vi "Bilateral_Filter.vi"() -> ()   [LabVIEW 2019]
doc: "This demo illustrates the grayscale morphological operations on grayscale images.\n\nOUTPUT:\nThe output of this demo displays the original grayscale image and the result of applying the grayscale morphological operation.\n\nSPECIAL EXAMPLES:\nSelect \"Images/Noisy-Images/Eggs-S&P90%.tif\" image for the following examples. This is an image corrupted by Salt and Pepper noise.\n\nDilation: Increasing the windows size from N=3 to N=25 increases peaks and decreases the size of valleys in the image. This is clear by seeing that the black noisy pixels vanish, while the white noisy pixels increase in size. The shape of the window can be seen at isolated white pixels illustrating an \"impulse reponse\" (try a cross shaped filter).\n\nErosion: Increasing the window size from N=3 to N=25 erodes/removes peaks (bright regions) and increases valleys (dark regions). The shape of the window can be seen at isolated dark pixels illustrating an \"impulse reponse\" (try a cross shaped filter).\n\nMedian (Majority): Possess attributes of both Dilation and Erosion operators - i.e. removes small black and white regions without changing the size of large objects. This option runs slower since the pixels have to be sorted first. \n\nClose: This operation removes small black objects, but does not change the size of the signal (like Dilation/Erosion). \n\nOpen: This operation removes small white objects, but does not change the size of the signal (like Dilation/Erosion).\n\nClose-Open (and Open-Close): This operation is very similar to the Median in its performance. However, there is an intense smoothing of the image, when compared to the Median filter."
uses:
  <vilib>/vision/NI_Vision_Development_Module.lvlib
panel:
  in  "SigmaS 2":dbl=1.0 format="%.2f"
  in  "sigma copy 2":dbl format="%.2f"
  in  "SigmaI":dbl=1.0 format="%.2f"
  in  "sigma copy":dbl format="%.2f"
  in  "SigmaS":dbl=1.0 format="%.2f"
  in  "STOP":bool
  in  "Window Shape copy":T1(ring)
  in  "Window Shape":T1(ring)
  in  "Save":bool
  in  "Zoom Facror copy":dbl=1.0 min=0.0 step=0.1 format="%.2f"
  in  "Zoom Factor":dbl=1.0 min=0.0 step=0.1 format="%.2f"
  in  "N copy":u8=3 min=3 max=25 step=2
  in  "N":u8=3 min=3 max=25 step=2
  in  "Read Image":bool
  out "test":u8
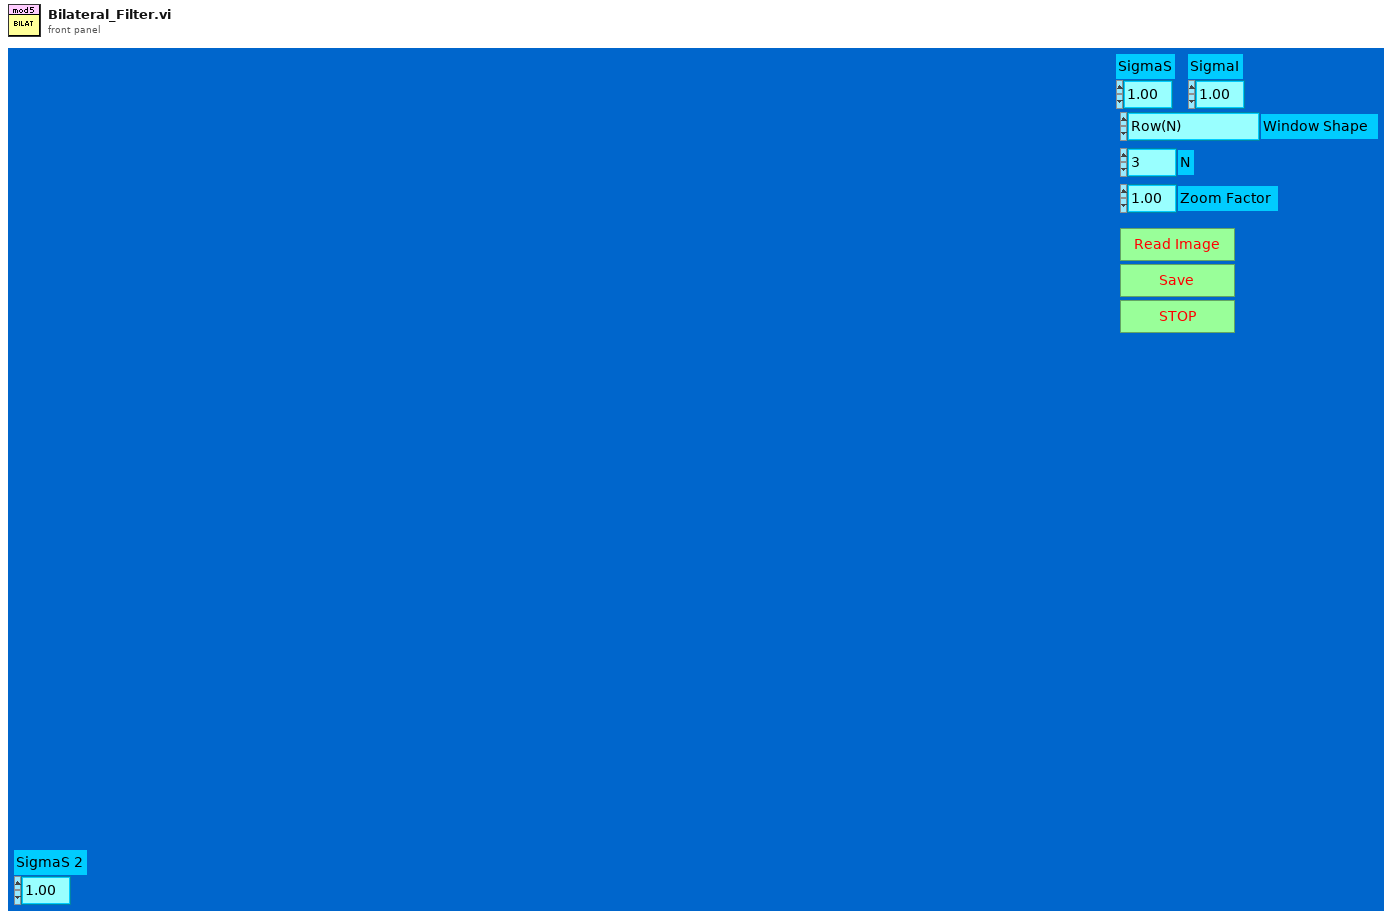
[diagram p1: front panel]
types:
  T1 = enum16{"Row(N)", "Col(N)", "Square(N^2)", "Cross(2N-1)", "XShape(2N-1)"}
  T2 = enum16{"No Operation", "Read Image", "Change BSize", "Compute Bilat", "Zoom Image", "Save Image"}
  T3 = enum16{"No Operation", "Read Image", "N Changed", "Compute Bilat", "Zoom Image", "Save Image"}
  T4 = typedef "IMAQ Image.ctl" = refnum<image>
  T5 = enum16{"existing file", "new file", "new or existing file", "existing dir", "new dir", "new or existing dir"}
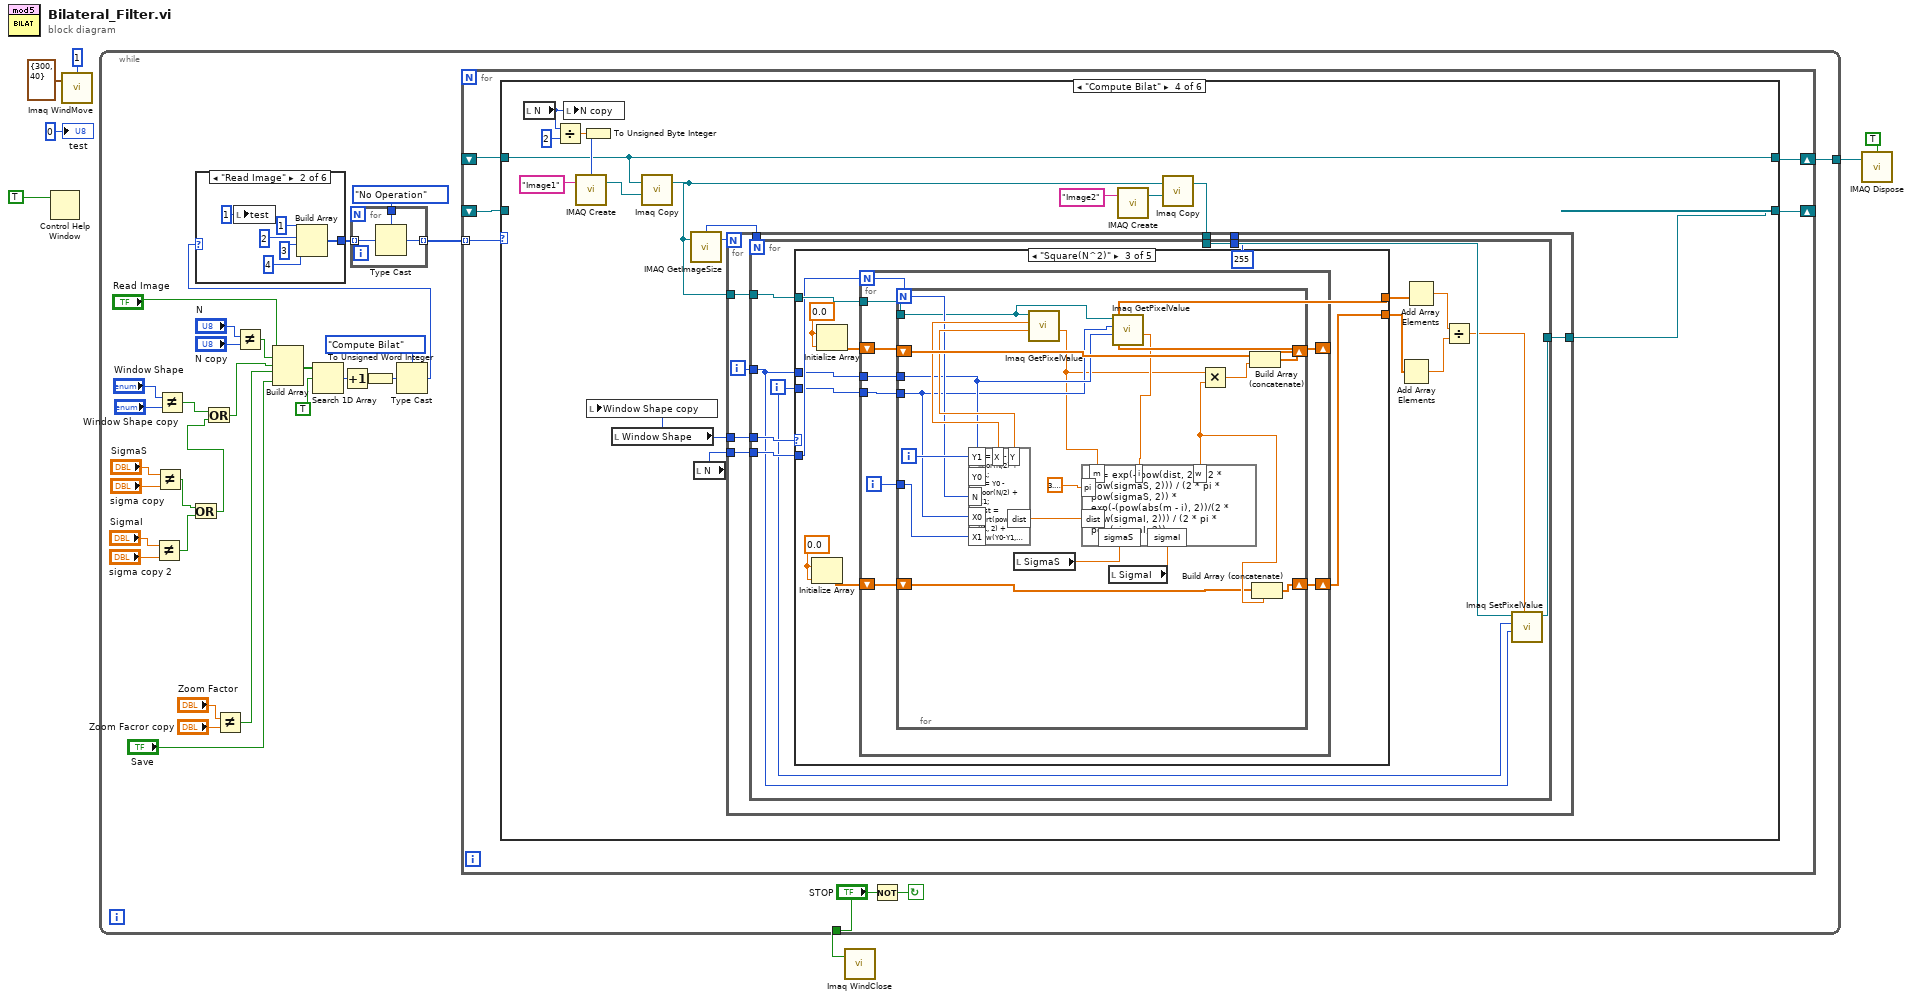
[diagram p0: block diagram]
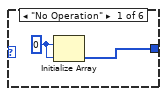
[diagram p2: hidden frame]
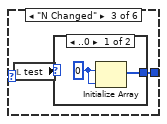
[diagram p3: hidden frame]
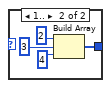
[diagram p4: hidden frame]
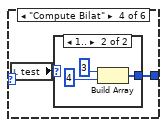
[diagram p5: hidden frame]
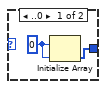
[diagram p6: hidden frame]
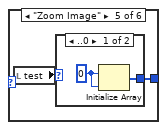
[diagram p7: hidden frame]
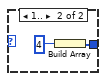
[diagram p8: hidden frame]
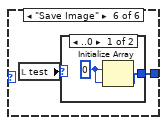
[diagram p9: hidden frame]
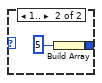
[diagram p10: hidden frame]
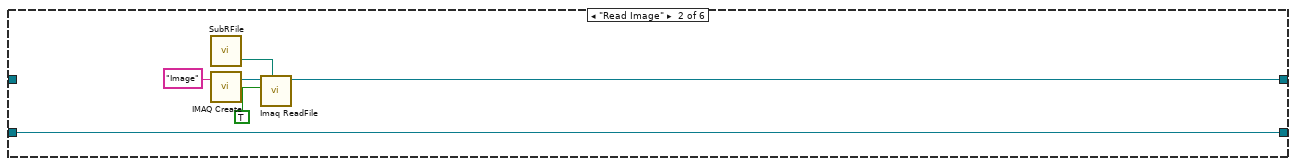
[diagram p12: hidden frame]
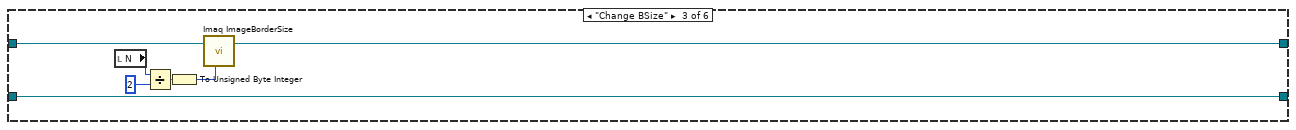
[diagram p13: hidden frame]
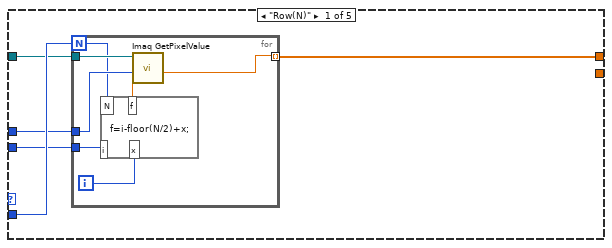
[diagram p14: hidden frame]
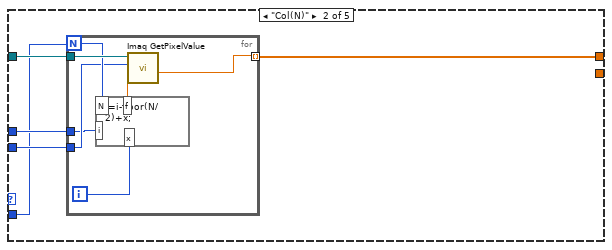
[diagram p15: hidden frame]
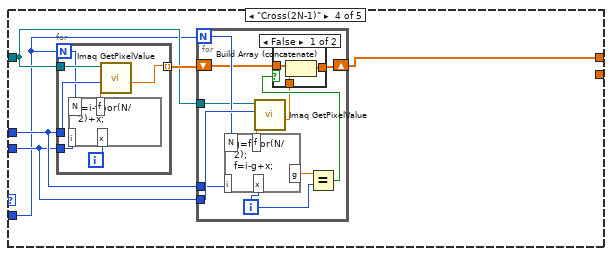
[diagram p16: hidden frame]
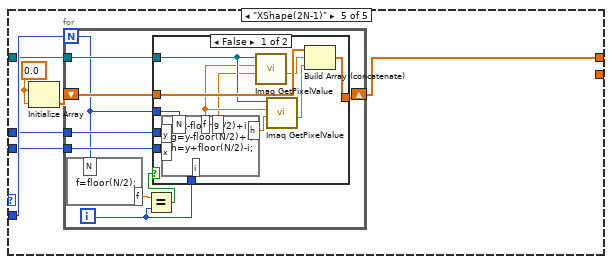
[diagram p18: hidden frame]
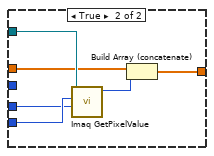
[diagram p19: hidden frame]
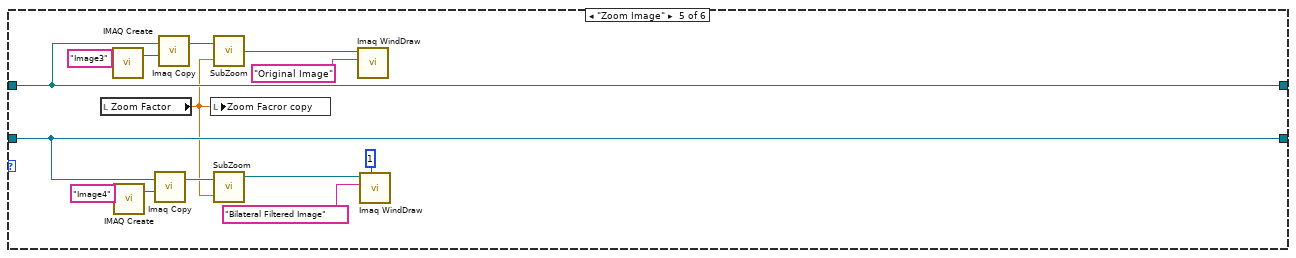
[diagram p20: hidden frame]
diagram:
  n1 = Control Help Window(1:TRUE ("Show")) -> ()  [unwired: 1 out]
  n2 = call "Imaq WindMove"("Window Number (0...15)"=1, "Coordinates (screen)"=cluster{"X Position":i32, "Y Position":i32} {"X Position"=300, "Y Position"=40}) -> ()  [unwired: 2 in, 3 out]
  n3 = while {
    tunnel: ["STOP"] -> w3
    tunnel: [w20] -> w5
    stop <- w38 continue-if-true
    n4 = Not Equal?(x="SigmaI", y="sigma copy 2") -> (x != y?=w9:bool)
    n5 = Not Equal?(x="SigmaS", y="sigma copy") -> (x != y?=w10:bool)
    n6 = Not Equal?(x="Window Shape", y="Window Shape copy") -> (x != y?=w14:bool)
    n7 = Or(x=w10, y=w9) -> (x .or. y?=w8:bool)
    n8 = Or(x=w14, y=w8) -> (x .or. y?=w13:bool)
    n9 = Not Equal?(x="Zoom Factor", y="Zoom Facror copy") -> (x != y?=w34:bool)
    n10 = Not Equal?(x="N", y="N copy") -> (x != y?=w29:bool)
    n11 = Build Array("Read Image", w29, w13, w34, "Save") -> (w33:bool[])
    n12 = Search 1D Array(1D array=w33, element=TRUE) -> (index of element=w31:i32)  [unwired: 1 out]
    n13 = Increment(x=w31) -> (x+1=w28:i32)
    n14 = To Unsigned Word Integer(number=w28) -> (unsigned 16bit integer=w27:u16)
    n15 = Type Cast(type=T3."Compute Bilat", x=w27) -> (*(type *) &x=w26:T3)
    n16 = case shown="\"Read Image\"" w26 {
      tunnel: [w43 w49 w52 w60 w67 w73] -> w25
      frame "No Operation" {
        w44 = u16 0
        n17 = Initialize Array(w44, w44) -> (w43:u16[])
      }
      frame "Read Image" {
        n18 = local write "test"(1) -> ()
        n19 = Build Array(u16 1, u16 2, u16 3, u16 4) -> (w49:u16[])
      }
      frame "N Changed" {
        n20 = local read "test"() -> (w51:u8)
        n21 = case shown="..0" w51 {
          tunnel: [w53 w56] -> w52
          frame ..0 {
            w54 = u16 0
            n22 = Initialize Array(w54, w54) -> (w53:u16[])
          }
          frame 1.. {
            n23 = Build Array(u16 2, u16 3, u16 4) -> (w56:u16[])
          }
        }
      }
      frame "Compute Bilat" {
        n24 = local read "test"() -> (w59:u8)
        n25 = case shown="1.." w59 {
          tunnel: [w61 w63] -> w60
          frame ..0 {
            w62 = u16 0
            n26 = Initialize Array(w62, w62) -> (w61:u16[])
          }
          frame 1.. {
            n27 = Build Array(u16 3, u16 4) -> (w63:u16[])
          }
        }
      }
      frame "Zoom Image" {
        n28 = local read "test"() -> (w66:u8)
        n29 = case shown="..0" w66 {
          tunnel: [w68 w70] -> w67
          frame ..0 {
            w69 = u16 0
            n30 = Initialize Array(w69, w69) -> (w68:u16[])
          }
          frame 1.. {
            n31 = Build Array(u16 4) -> (w70:u16[])
          }
        }
      }
      frame "Save Image" {
        n32 = local read "test"() -> (w72:u8)
        n33 = case shown="..0" w72 {
          tunnel: [w74 w76] -> w73
          frame ..0 {
            w75 = u16 0
            n34 = Initialize Array(w75, w75) -> (w74:u16[])
          }
          frame 1.. {
            n35 = Build Array(u16 5) -> (w76:u16[])
          }
        }
      }
    }
    n36 = for {
      tunnel: w25 -> [w42] mode=indexing
      tunnel: [w41] -> w24 mode=indexing
      tunnel: T2."No Operation" -> [w40]
      n37 = Type Cast(type=w40, x=w42) -> (*(type *) &x=w41:T2)
    }
    n38 = for {
      tunnel: w24 -> [w78] mode=indexing
      shift-right: [w82] -> _
      shift-left: _ -> [w81]
      shift-right: [w80] -> w20
      shift-left: _ -> [w79]
      n39 = case shown="\"Compute Bilat\"" w78 {
        tunnel: w79 -> [w84 _ w97 w99 w265 w276]
        tunnel: [w84 w86 w96 w99 w265 w276] -> w80
        tunnel: [w83 w85 w95 w98 w263 w275] -> w82
        tunnel: w81 -> [w83 w85 w95 _ w263 w275]
        frame "No Operation" {
        }
        frame "Read Image" {
          n40 = call "SubRFile.vi"() -> ("selected file"=w88:path)  [unwired: 2 in, 1 out]
          n41 = call "IMAQ Create"("Image Name"="Image") -> ("New Image"=w89:T4)  [unwired: 3 in, 2 out]
          n42 = call "Imaq ReadFile"("File Path"=w88, "Load Color Palette? (No)"=TRUE, "Image"=w89) -> ("Image Out"=w86:T4)  [unwired: 2 in, 6 out]
        }
        frame "Change BSize" {
          n43 = local read "N"() -> (w94:u8)
          n44 = Divide(x=w94, y=u8 2) -> (x/y=w92:dbl)
          n45 = To Unsigned Byte Integer(number=w92) -> (unsigned 8bit integer=w91:u8)
          n46 = call "Imaq ImageBorderSize"("Image"=w97, "Image border size in"=w91) -> ("Image Out"=w96:T4)  [unwired: 2 in, 2 out]
        }
        frame "Compute Bilat" {
          n47 = local read "N"() -> (w102:u8)
          n48 = Divide(x=w102, y=u8 2) -> (x/y=w111:dbl)
          n49 = local write "N copy"(w102) -> ()
          n50 = To Unsigned Byte Integer(number=w111) -> (unsigned 8bit integer=w109:u8)
          n51 = call "IMAQ Create"("Border Size"=w109, "Image Name"="Image1") -> ("New Image"=w100:T4)  [unwired: 2 in, 2 out]
          n52 = local read "Window Shape"() -> (w113:T1)
          n53 = local write "Window Shape copy"(w113) -> ()
          n54 = call "Imaq Copy"("Image Dst"=w100, "Image Src"=w99) -> ("Image Dst Out"=w101:T4)  [unwired: 4 in, 1 out]
          n55 = call "IMAQ GetImageSize"("Image"=w101) -> ("Y Resolution"=w108:i32, "X Resolution"=w106:i32)  [unwired: 1 in, 3 out]
          n56 = local read "N"() -> (w103:u8)
          n57 = call "IMAQ Create"("Image Name"="Image2") -> ("New Image"=w105:T4)  [unwired: 3 in, 2 out]
          n58 = call "Imaq Copy"("Image Dst"=w105, "Image Src"=w101) -> ("Image Dst Out"=w107:T4)  [unwired: 1 in, 4 out]
          n59 = for {
            N: w108 -> [_]
            tunnel: w106 -> [w121]
            tunnel: w113 -> [w120]
            tunnel: w103 -> [w119]
            tunnel: w107 -> [w117]
            tunnel: [w116] -> w98
            tunnel: [w115] -> _
            tunnel: w101 -> [w114]
            i -> [w118]
            n60 = for {
              N: w121 -> [_]
              tunnel: w114 -> [w132]
              tunnel: w120 -> [w134]
              tunnel: w119 -> [w133]
              tunnel: w118 -> [w130]
              tunnel: w117 -> [w129]
              tunnel: [w128] -> w116
              tunnel: [255] -> w115
              i -> [w131]
              n61 = case shown="\"Square(N^2)\"" w134 {
                tunnel: w133 -> [w139 w148 w166 w198 w232]
                tunnel: w132 -> [w138 w151 w167 w199 w231]
                tunnel: w130 -> [w137 w150 w163 w201 w227]
                tunnel: w131 -> [w136 w149 w162 w200 w226]
                tunnel: [w135 w147 w164 w202 w228] -> w125
                tunnel: [_ _ w159 _ _] -> w126
                frame "Row(N)" {
                  n62 = for {
                    N: w139 -> [w142]
                    tunnel: w138 -> [w146]
                    tunnel: w137 -> [w145]
                    tunnel: w136 -> [w143]
                    tunnel: [w140] -> w135 mode=indexing
                    i -> [w141]
                    n63 = formula code="f=i-floor(N/2)+x;"("i"=w143, "x"=w141, "N"=w142) -> ("f"=w144:dbl)
                    n64 = call "Imaq GetPixelValue"("Image"=w146, "X Coordinate"=w144, "Y Coordinate"=w145) -> ("Pixel Value (Float)"=w140:sgl)  [unwired: 1 in, 6 out]
                  }
                }
                frame "Col(N)" {
                  n65 = for {
                    N: w148 -> [w157]
                    tunnel: w151 -> [w158]
                    tunnel: w150 -> [w153]
                    tunnel: w149 -> [w155]
                    tunnel: [w152] -> w147 mode=indexing
                    i -> [w156]
                    n66 = formula code="f=i-floor(N/2)+x;"("i"=w153, "x"=w156, "N"=w157) -> ("f"=w154:dbl)
                    n67 = call "Imaq GetPixelValue"("Image"=w158, "X Coordinate"=w155, "Y Coordinate"=w154) -> ("Pixel Value (Float)"=w152:sgl)  [unwired: 1 in, 6 out]
                  }
                }
                frame "Square(N^2)" {
                  w161 = sgl 0.0
                  w168 = sgl 0.0
                  n68 = Initialize Array(w161, w161) -> (w160:sgl[])
                  n69 = Initialize Array(w168, w168) -> (w165:sgl[])
                  n70 = for {
                    N: w166 -> [w173]
                    tunnel: w167 -> [w177]
                    shift-right: [w175] -> w164
                    shift-left: w165 -> [w176]
                    tunnel: w163 -> [w172]
                    tunnel: w162 -> [w174]
                    shift-right: [w169] -> w159
                    shift-left: w160 -> [w170]
                    i -> [w171]
                    n71 = for {
                      N: w173 -> [w191]
                      tunnel: w177 -> [w188]
                      shift-right: [w196] -> w175
                      shift-left: w176 -> [w197]
                      tunnel: w174 -> [w189]
                      tunnel: w172 -> [w190]
                      tunnel: w171 -> [w194]
                      shift-right: [w178] -> w169
                      shift-left: w170 -> [w179]
                      i -> [w195]
                      n72 = formula code="X = X0 - floor(N/2) + X1;\nY = Y0 - floor(N/2) + X1;\ndist = sqrt(pow(X0-X1, 2) + pow(Y0-Y1, 2));"("Y1"=w195, "X1"=w194, "X0"=w189, "Y0"=w190, "N"=w191) -> ("X"=w193:dbl, "Y"=w192:dbl, "dist"=w186:dbl)
                      n73 = local read "SigmaS"() -> (w182:dbl)
                      n74 = call "Imaq GetPixelValue"("Image"=w188, "X Coordinate"=w193, "Y Coordinate"=w192) -> ("Pixel Value (Float)"=w183:sgl)  [unwired: 1 in, 6 out]
                      n75 = local read "SigmaI"() -> (w181:dbl)
                      n76 = call "Imaq GetPixelValue"("Image"=w188, "X Coordinate"=w189, "Y Coordinate"=w190) -> ("Pixel Value (Float)"=w187:sgl)  [unwired: 1 in, 6 out]
                      n77 = formula code="w = exp(-(pow(dist, 2))/(2 * pow(sigmaS, 2))) / (2 * pi * pow(sigmaS, 2)) * exp(-(pow(abs(m - i), 2))/(2 * pow(sigmaI, 2))) / (2 * pi * pow(sigmaI, 2));"("m"=w183, "i"=w187, "dist"=w186, "pi"=3.141592653589793, "sigmaS"=w182, "sigmaI"=w181) -> ("w"=w180:dbl)
                      n78 = Multiply(x=w183, y=w180) -> (x*y=w184:dbl)
                      n79 = Build Array (concatenate)(w197, w184) -> (w196:dbl[])
                      n80 = Build Array (concatenate)(w179, w180) -> (w178:dbl[])
                    }
                  }
                }
                frame "Cross(2N-1)" {
                  n81 = for {
                    N: w198 -> [w221]
                    tunnel: w199 -> [w225]
                    tunnel: w201 -> [w224]
                    tunnel: w200 -> [w222]
                    tunnel: [w219] -> w203 mode=indexing
                    i -> [w220]
                    n82 = formula code="f=i-floor(N/2)+x;"("i"=w222, "x"=w220, "N"=w221) -> ("f"=w223:dbl)
                    n83 = call "Imaq GetPixelValue"("Image"=w225, "X Coordinate"=w223, "Y Coordinate"=w224) -> ("Pixel Value (Float)"=w219:sgl)  [unwired: 1 in, 6 out]
                  }
                  n84 = for {
                    N: w198 -> [w210]
                    shift-right: [w208] -> w202
                    shift-left: w203 -> [w209]
                    tunnel: w201 -> [w211]
                    tunnel: w200 -> [w212]
                    tunnel: w199 -> [w207]
                    i -> [w214]
                    n85 = formula code="g=floor(N/2);\nf=i-g+x;"("i"=w211, "x"=w214, "N"=w210) -> ("f"=w213:dbl, "g"=w206:dbl)
                    n86 = call "Imaq GetPixelValue"("Image"=w207, "X Coordinate"=w212, "Y Coordinate"=w213) -> ("Pixel Value (Float)"=w204:sgl)  [unwired: 1 in, 6 out]
                    n87 = Equal?(x=w206, y=w214) -> (x = y?=w205:bool)
                    n88 = case shown="False" w205 {
                      tunnel: w204 -> [w217 _]
                      tunnel: [w216 w218] -> w208
                      tunnel: w209 -> [w215 w218]
                      frame False {
                        n89 = Build Array (concatenate)(w215, w217) -> (w216:sgl[])
                      }
                      frame True {
                      }
                    }
                  }
                }
                frame "XShape(2N-1)" {
                  w230 = sgl 0.0
                  n90 = Initialize Array(w230, w230) -> (w229:sgl[])
                  n91 = for {
                    N: w232 -> [w233]
                    tunnel: w231 -> [w236]
                    shift-right: [w235] -> w228
                    shift-left: w229 -> [w239]
                    tunnel: w227 -> [w238]
                    tunnel: w226 -> [w237]
                    i -> [w234]
                    n92 = formula code="f=floor(N/2);"("N"=w233) -> ("f"=w241:dbl)
                    n93 = Equal?(x=w241, y=w234) -> (x = y?=w240:bool)
                    n94 = case shown="False" w240 {
                      tunnel: w239 -> [w253 w256]
                      tunnel: w238 -> [w250 w257]
                      tunnel: w237 -> [w249 w259]
                      tunnel: w236 -> [w251 w258]
                      tunnel: [w252 w254] -> w235
                      tunnel: w234 -> [w248 _]
                      tunnel: w233 -> [w247 _]
                      frame False {
                        n95 = formula code="f=x-floor(N/2)+i;\ng=y-floor(N/2)+i;\nh=y+floor(N/2)-i;"("y"=w250, "x"=w249, "i"=w248, "N"=w247) -> ("f"=w246:dbl, "g"=w245:dbl, "h"=w244:dbl)
                        n96 = call "Imaq GetPixelValue"("Image"=w251, "X Coordinate"=w246, "Y Coordinate"=w245) -> ("Pixel Value (Float)"=w242:sgl)  [unwired: 1 in, 6 out]
                        n97 = call "Imaq GetPixelValue"("Image"=w251, "X Coordinate"=w246, "Y Coordinate"=w244) -> ("Pixel Value (Float)"=w243:sgl)  [unwired: 1 in, 6 out]
                        n98 = Build Array (concatenate)(w253, w242, w243) -> (w252:sgl[])
                      }
                      frame True {
                        n99 = call "Imaq GetPixelValue"("Image"=w258, "X Coordinate"=w259, "Y Coordinate"=w257) -> ("Pixel Value (U8)"=w255:u8)  [unwired: 1 in, 6 out]
                        n100 = Build Array (concatenate)(w256, w255) -> (w254:sgl[])
                      }
                    }
                  }
                }
              }
              n101 = Add Array Elements(numeric array=w126) -> (sum=w123:dbl)
              n102 = Add Array Elements(numeric array=w125) -> (sum=w124:dbl)
              n103 = Divide(x=w124, y=w123) -> (x/y=w122:dbl)
              n104 = call "Imaq SetPixelValue"("Pixel Value"=w122, "Y Coordinate"=w130, "X Coordinate"=w131, "Image"=w129) -> ("Image Out"=w128:T4)  [unwired: 1 in, 6 out]
            }
          }
        }
        frame "Zoom Image" {
          n105 = local read "Zoom Factor"() -> (w262:dbl)
          n106 = call "IMAQ Create"("Image Name"="Image3") -> ("New Image"=w271:T4)  [unwired: 3 in, 2 out]
          n107 = call "IMAQ Create"("Image Name"="Image4") -> ("New Image"=w268:T4)  [unwired: 3 in, 2 out]
          n108 = call "Imaq Copy"("Image Dst"=w268, "Image Src"=w263) -> ("Image Dst Out"=w269:T4)  [unwired: 1 in, 4 out]
          n109 = call "Imaq Copy"("Image Dst"=w271, "Image Src"=w265) -> ("Image Dst Out"=w272:T4)  [unwired: 1 in, 4 out]
          n110 = local write "Zoom Facror copy"(w262) -> ()
          n111 = call "SubZoom.vi"("Factor"=w262, "Image Src"=w272) -> ("Image Dst Out"=w266:T4)
          n112 = call "SubZoom.vi"("Factor"=w262, "Image Src"=w269) -> ("Image Dst Out"=w264:T4)
          n113 = call "Imaq WindDraw"("Title"="Original Image", "Image"=w266) -> ()  [unwired: 4 in, 6 out]
          n114 = call "Imaq WindDraw"("Window Number (0...15)"=1, "Title"="Bilateral Filtered Image", "Image"=w264) -> ()  [unwired: 3 in, 6 out]
        }
        frame "Save Image" {
          (unwired) T5."new or existing file" ("select mode (2)")
          n115 = File Dialog(7:"Enter the name of the file you want to  Save  " ("prompt")) -> (0:w274:errorcluster, 3:w277:path)  [unwired: 1 in, 7 out]
          n116 = Unbundle(w274) -> ()  [unwired: 3 out]
          n117 = call "Imaq WriteFile"("File Type"="TIFF", "File Path"=w277, "Image"=w275) -> ()  [unwired: 2 in, 4 out]
        }
      }
    }
    n118 = Not(x="STOP") -> (.not. x?=w38:bool)
  }
  n119 = call "Imaq WindClose"("Close All Windows (False)"=w3) -> ()  [unwired: 2 in, 4 out]
  n120 = call "IMAQ Dispose"("All Images? (No)"=TRUE, "Image"=w5) -> ()  [unwired: 1 in, 4 out]
  "test" <- 0
